vi "gatherTrunkVars.vi"() -> (0 "BoundaryYtrunk":dbl[](array[numeric]), 1 "BoundaryXtrunk":dbl[](array[numeric]), 2 "trunkCen":dbl[](array[numeric]), 3 "viconData":dbl[](array[numeric]), 4 "Fdesired":dbl, 8 "FM --- FF":dbl[](array[numeric]))   [LabVIEW 2017]
panel:
  # "Pelvis Variables for FF"
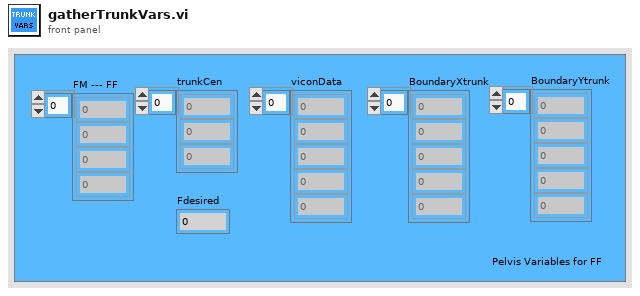
[diagram p1: front panel]
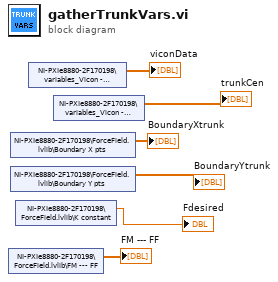
[diagram p0: block diagram]
diagram:
  n1 = shared-variable "NI-PXIe8880-2F170198\\ForceField.lvlib\\FM --- FF"() -> (→"FM --- FF":dbl[])  [unwired: 1 in, 1 out]
  n2 = shared-variable "NI-PXIe8880-2F170198\\ForceField.lvlib\\Boundary X pts"() -> (→"BoundaryXtrunk":dbl[])  [unwired: 1 in, 1 out]
  n3 = shared-variable "NI-PXIe8880-2F170198\\ForceField.lvlib\\Boundary Y pts"() -> (→"BoundaryYtrunk":dbl[])  [unwired: 1 in, 1 out]
  n4 = shared-variable "NI-PXIe8880-2F170198\\ForceField.lvlib\\K constant"() -> (→"Fdesired":dbl)  [unwired: 1 in, 1 out]
  n5 = shared-variable "NI-PXIe8880-2F170198\\variables_Vicon - networkPublished.lvlib\\viconData"() -> (→"viconData":dbl[])  [unwired: 1 in, 1 out]
  n6 = shared-variable "NI-PXIe8880-2F170198\\variables_Vicon - networkPublished.lvlib\\trunk_cn"() -> (→"trunkCen":dbl[])  [unwired: 1 in, 1 out]
